vi "HMI.vi"(8 "error in (no error)":errorcluster caption="entrée d'erreur (pas d'erreur)", 11 "Class Popup WaitDIO en entrée":refnum<class "Class Popup WaitWeight.lvclass">) -> (0 "error out":errorcluster caption="sortie d'erreur", 1 "Input":string, 2 "Operator_Selection":bool, 3 "Class Popup WaitDIO en sortie":refnum<class "Class Popup WaitWeight.lvclass">)   [LabVIEW 2020, in "Library Instrument & Equipement.lvlib" / "Library Popup.lvlib" / "Class Popup WaitWeight.lvclass"]
uses:
  Class Popup WaitWeight.lvclass
  C:/Users/ngarcin/OneDrive - Altyor/Standard TB/Class/Popup/Class Popup (Main)/Class Popup (Main).lvclass
  C:/Users/ngarcin/OneDrive - Altyor/Standard TB/Class/Popup/Class Popup Operator_Validation/Class Popup Operator_Validation (Default)/Class Popup Operator_Validation (Virtual).lvclass
  Commun VI/TypeDef/Liste Error.ctl
  JSON API/JSON Value/Set from JSON string.vi
  Instrument/Instrument (Default)/Class Instrument (Default).lvclass
  JSON API/JSON Value/JSON Value.lvclass
  Class Popup Operator_Validation/Class Popup Operator_Validation (Default)/Class Popup Operator_Validation (Virtual).lvclass
  Class Popup WaitWeight.lvclass/Class Popup WaitWeight.ctl
  JSON API/Variant JSON/Variant JSON.lvlib
  JSON API/Get Polymorphic/JSON GetSet.lvlib
  Commun VI/Library Commun.lvlib
panel:
  out "Json_String":string
  out "Image":picture
  out "Text":string
  in  "Bouton NOK":bool caption="Default"
  in  "Bouton OK":bool caption="Validated"
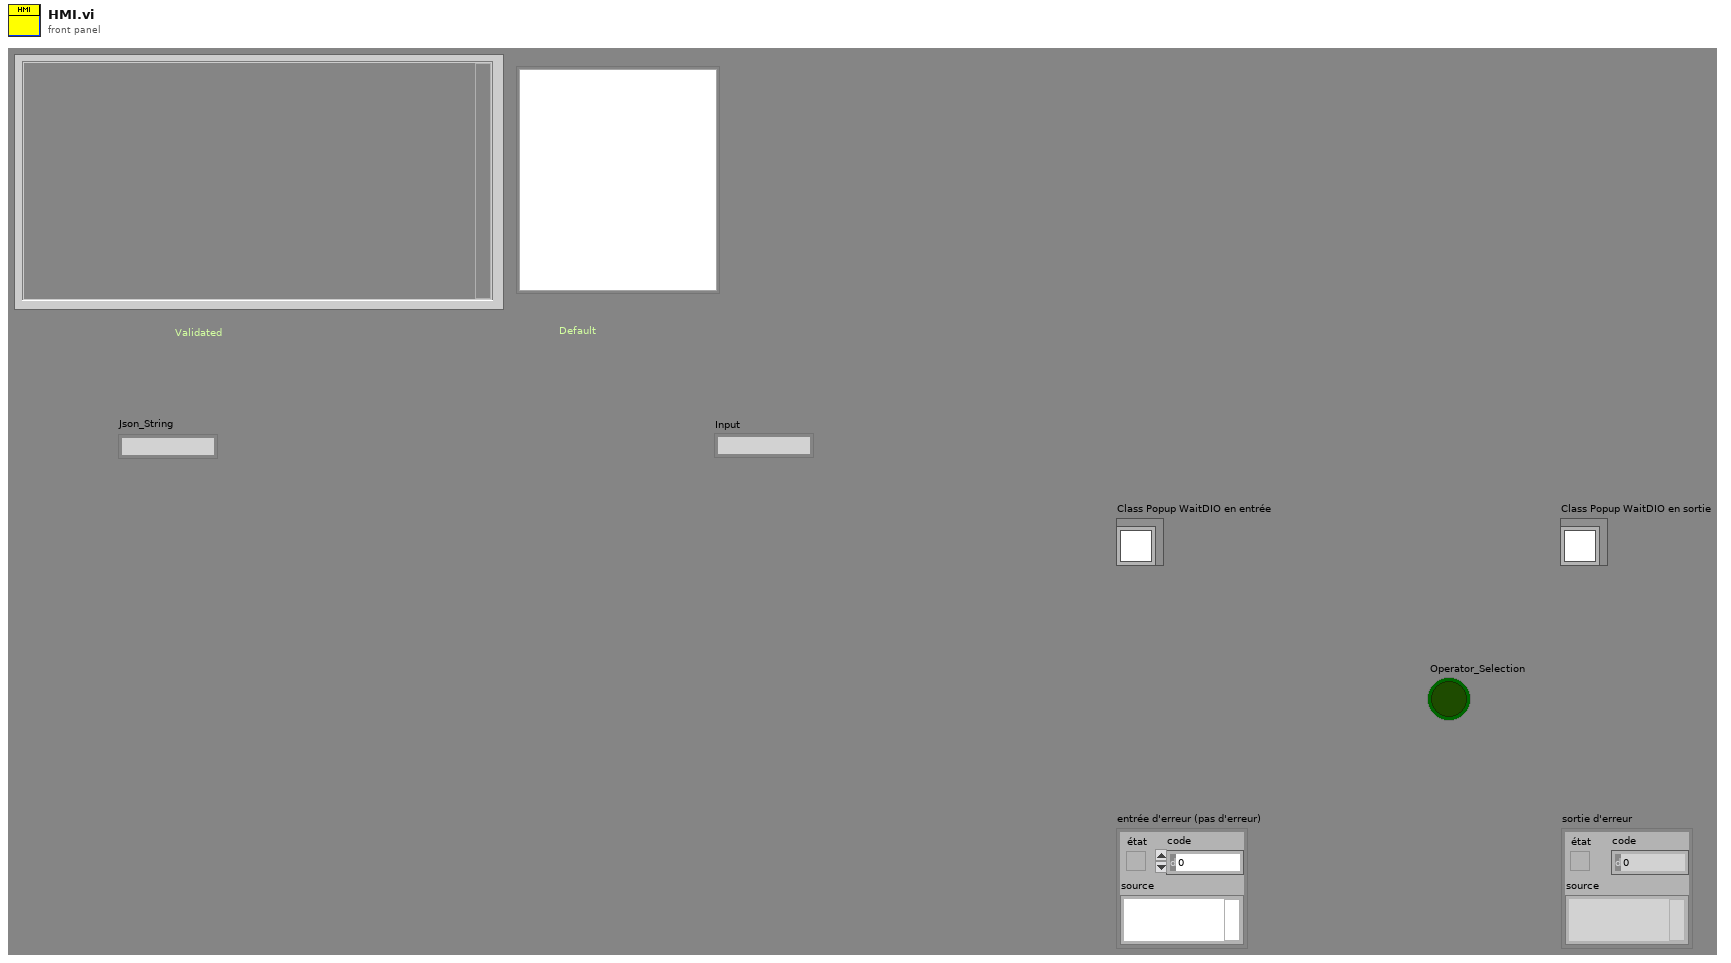
[diagram p1: front panel]
types:
  T1 = cluster{"Instrument":refnum<class "Class Instrument (Default).lvclass">, "Timeout (ms)":u64, "Weight":dbl, "Front":enum16{"Amount", "Descending"}}
  T2 = typedef "Library Commun.lvlib/Liste Error.ctl" = enum16{"Firebase Driver - Get Document", "Firebase Driver - Get Document With Where", "Firebase Driver - Delete Document", "Firebase Driver - Set Document", "Firebase Driver - Update Document", "Firebase Altyor - Search Document Bench", "Firebase Altyor - Class Not in Firebase", "Spectrum_Analyser - Timeout", "Relay Board - Qty Relay", "DIO - Pb Funtion", "Power_Supply - Peripherical not find", "Mutimeter - Peripherical not find", "Instrument - Function Not Used", "Instrument - Instrument name not specified", "Instrument - Allready Initialised", "Instrument - TimeOut", "Instrument - the instrument must be Initialise before", "Instrument - Frame Not received", "Instrument - Frame Nok", "Test - Initialise the File_for_Save", "Test - Timeout", "Test - Cmd Error", "FGV - Variable ", "BDD FireBase - Define Class", "SN - Class Not Define"}
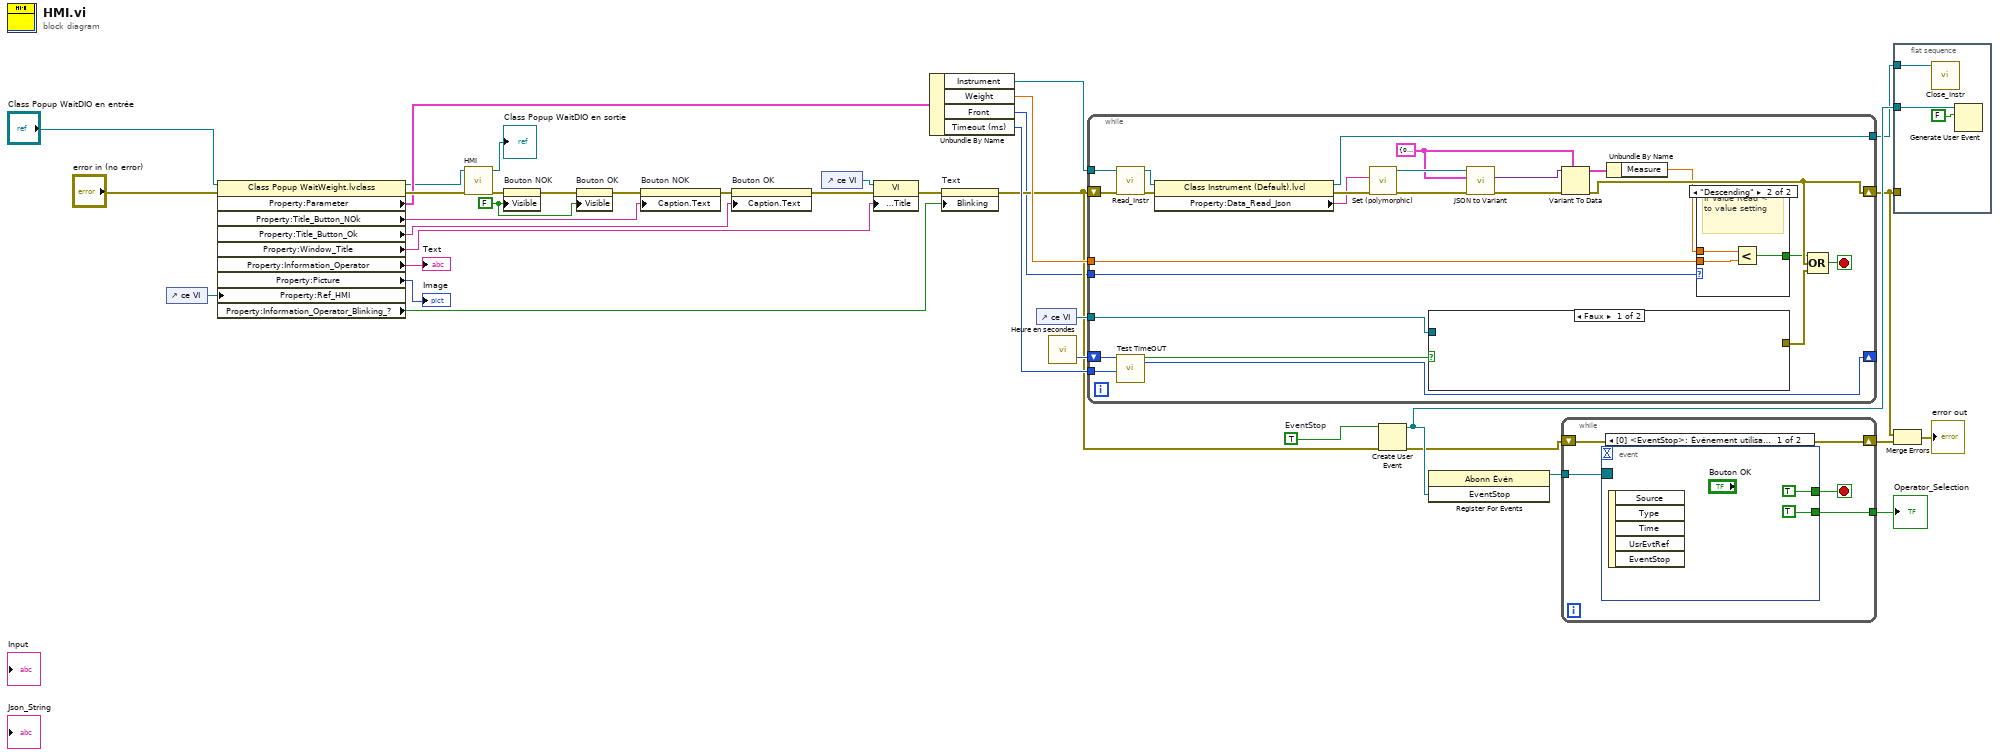
[diagram p0: block diagram]
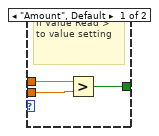
[diagram p2: hidden frame]
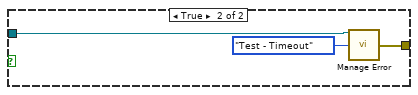
[diagram p3: hidden frame]
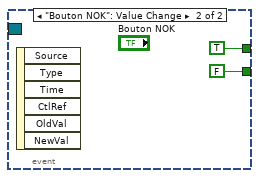
[diagram p4: hidden frame]
diagram:
  w19 = TRUE  # EventStop
  w23 = FALSE ("Visible")
  n1 = control-ref of="ce VI"() -> (w28:refnum<vi>)
  n2 = property class="Class Popup WaitWeight.lvclass"(reference="Class Popup WaitDIO en entrée", error in="error in (no error)", "Property:Ref_HMI"=w28) -> (reference out=w3:refnum<class "Class Popup WaitWeight.lvclass">, error out=w12:errorcluster, "Property:Parameter"=w5:T1, "Property:Title_Button_NOk"=w36:string, "Property:Title_Button_Ok"=w37:string, "Property:Window_Title"=w31:string, "Property:Information_Operator"=→"Text":string, "Property:Picture"=→"Image":picture, "Property:Information_Operator_Blinking_?"=w26:bool)
  n3 = call-parent "HMI.vi"("error in (no error)"=w12, "Class Popup Operator_Validation (Default) en entrée"=w3) -> ("error out"=w4:errorcluster, "Class Popup Operator_Validation (Default) en sortie"=→"Class Popup WaitDIO en sortie":refnum<class "Class Popup WaitWeight.lvclass">)  [unwired: 6 in, 2 out]
  n4 = property on="Bouton NOK" class="Bool"(error in=w4, "Visible"=w23) -> (error out=w35:errorcluster)  [unwired: 1 in, 1 out]
  n5 = property on="Bouton OK" class="Bool"(error in=w35, "Visible"=w23) -> (error out=w34:errorcluster)  [unwired: 1 in, 1 out]
  n6 = property on="Bouton NOK" class="Bool"(error in=w34, "Caption.Text"=w36) -> (error out=w33:errorcluster)  [unwired: 1 in, 1 out]
  n7 = property on="Bouton OK" class="Bool"(error in=w33, "Caption.Text"=w37) -> (error out=w11:errorcluster)  [unwired: 1 in, 1 out]
  n8 = control-ref of="ce VI"() -> (w32:refnum<vi>)
  n9 = property class="VI"(reference=w32, error in=w11, "Front Panel.Title"=w31) -> (error out=w27:errorcluster)  [unwired: 1 out]
  n10 = Unbundle By Name(w5) -> ("Instrument"=w8:refnum<class "Class Instrument (Default).lvclass">, "Weight"=w13:dbl, "Front"=w1:enum16{"Amount", "Descending"}, "Timeout (ms)"=w14:u64)
  n11 = property on="Text" class="Ch"(error in=w27, "Blinking"=w26) -> (error out=w7:errorcluster)  [unwired: 1 in, 1 out]
  n12 = control-ref of="ce VI"() -> (w21:refnum<vi>)
  n13 = call "Heure en secondes.vi"() -> ("Heure en milisecondes"=w22:u32)  [unwired: 2 in, 1 out]
  n14 = while {
    tunnel: w8 -> [w62]
    shift-right: [w52] -> w15
    shift-left: w7 -> [w61]
    tunnel: w14 -> [w48]
    shift-right: [w49] -> _
    shift-left: w22 -> [w50]
    tunnel: w21 -> [w47]
    tunnel: w13 -> [w40]
    tunnel: [w44] -> w9
    tunnel: w1 -> [w38]
    stop <- w51 stop-if-true
    w43 = cluster{"Measure":dbl, "In_TimeOut":bool} {"Measure"=0.0, "In_TimeOut"=FALSE}
    n15 = call-dynamic "Read_Instr.vi"("error in (no error)"=w61, "Class Instrument (Default) en entrée"=w62) -> ("error out"=w53:errorcluster, "Class Instrument (Default) en sortie"=w60:refnum<class "Class Instrument (Default).lvclass">)  [unwired: 8 in]
    n16 = call "Test TimeOUT.vi"("OLD Time"=w50, "TimeOut ms"=w48) -> ("Timeout ?"=w46:bool, "NEW Time"=w49:u32)  [unwired: 13 in, 3 out]
    n17 = property class="Class Instrument (Default).lvcl"(reference=w60, error in=w53) -> (reference out=w44:refnum<class "Class Instrument (Default).lvclass">, error out=w55:errorcluster, "Property:Data_Read_Json"=w54:string)
    n18 = call-poly "Set (polymorphic).vi"("error in (no error)"=w55, "JSON stream"=w54) -> ("error out"=w58:errorcluster, "JSON Value out"=w56:refnum<class "JSON Value.lvclass">)  [unwired: 7 in, 1 out]
    n19 = case shown="Faux" w46 {
      tunnel: w47 -> [_ w70]
      tunnel: [_ w69] -> w45
      frame False {
      }
      frame True {
        n20 = call "Manage Error.vi"("VI in Error"=w70, "Code Erreur"=Liste_Error."Test - Timeout") -> ("error out"=w69:errorcluster)  [unwired: 13 in]
      }
    }
    n21 = call "JSON to Variant.vi"("error in (no error)"=w58, "Variant (Data Type)"=w43, "JSON Value"=w56) -> ("error out"=w57:errorcluster, "Variant out"=w59:variant)  [unwired: 7 in]
    n22 = Variant To Data(error in=w57, type=w43, Variant=w59) -> (data=w42:cluster{"Measure":dbl, "In_TimeOut":bool}, error out=w52:errorcluster)
    n23 = Unbundle By Name(w42) -> ("Measure"=w41:dbl)
    n24 = case shown="\"Descending\"" w38 {
      tunnel: w41 -> [w65 w68]
      tunnel: w40 -> [w64 w67]
      tunnel: [w63 w66] -> w39
      frame "Amount", Default {
        # "If Value Read > to value setting"
        n25 = Greater?(x=w65, y=w64) -> (0:w63:bool)
      }
      frame "Descending" {
        # "If Value Read < to value setting"
        n26 = Less?(x=w68, y=w67) -> (x < y?=w66:bool)
      }
    }
    n27 = Compound Arithmetic op=OR ("Opérateur arithmétique")(w39, w52, w45) -> (w51:bool)
  }
  n28 = Create User Event(user event datatype=w19, error in=w7) -> (user event=w18:refnum<user-event>, error out=w10:errorcluster)
  n29 = register-events(w18) -> (reference out=w20:refnum<event-registration>)  [unwired: 2 in, 1 out]
  n30 = while {
    tunnel: [w73] -> w24
    shift-right: [w74] -> w16
    shift-left: w10 -> [w74]
    tunnel: w20 -> [w72]
    stop <- w75 stop-if-true
    n31 = event shown="[0] <EventStop>: Événement utilisateur" {
      selector: w72 -> [_ _]
      dyn-events: _ -> [_ _]
      timeout: _ -> [_ _]
      tunnel: [TRUE ("Valeur (Signalisation)") TRUE ("Valeur (Signalisation)")] -> w75
      tunnel: [TRUE ("Operator_Selection") FALSE ("Operator_Selection")] -> w73
      event User Event {
        n32 = event-data() -> ()  [unwired: 1 in, 5 out]
      }
      event "Bouton NOK": Value Change {
        n33 = event-data() -> ()  [unwired: 1 in, 6 out]
      }
    }
  }
  "Operator_Selection" <- w24
  n34 = flat-sequence {
    tunnel: w18 -> [w82]
    tunnel: w15 -> [_]
    tunnel: w9 -> [w80]
    frame #0 {
      n35 = call-dynamic "Close_Instr.vi"("Class Instrument (Default) en entrée"=w80) -> ()  [unwired: 9 in, 2 out]
      n36 = Generate User Event(user event=w82, event data cluster=FALSE ("données d'événement")) -> ()  [unwired: 2 in, 2 out]
    }
  }
  n37 = Merge Errors(w15, w16) -> (→"error out":errorcluster)
